vi "Get Step by Index.vi"(8 "error in (no error)":errorcluster, 10 "Step Index":i32, 11 "Sequence in":refnum<class "Sequence.lvclass">) -> (0 "error out":errorcluster, 2 "Step":refnum<class "Step.lvclass">, 3 "Sequence out":refnum<class "Sequence.lvclass">)   [LabVIEW 2020, in "Tester.lvlib" / "Sequence.lvclass"]
uses:
  Sequence.lvclass
  Step/Step.lvclass
  Sequence.lvclass/Sequence.ctl
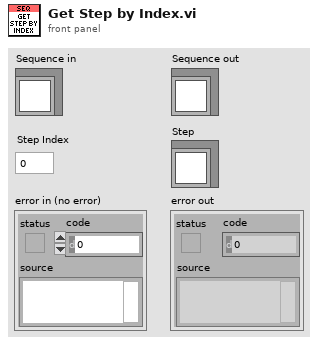
[diagram p1: front panel]
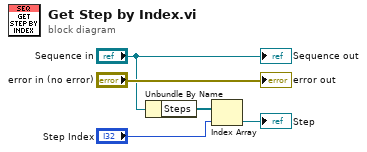
[diagram p0: block diagram]
diagram:
  n1 = Unbundle By Name("Sequence in") -> ("Steps"=w3:refnum<class "Step.lvclass">[])
  n2 = Index Array(array=w3, index="Step Index") -> (element=→"Step":refnum<class "Step.lvclass">)
  "error out" <- "error in (no error)"
  "Sequence out" <- "Sequence in"
